vi "NEW LOAD CELL PID.vi"(5 "filtered_load_in":dbl, 6 "filtered_deriv_in":dbl, 7 "integral_out":dbl, 8 "error in (no error)":errorcluster, 9 "prev_error_out":dbl, 10 "Checkbox":bool, 11 "main ref":T1) -> (0 "error out":errorcluster, 1 "prev_error_out":dbl, 2 "integral_out":dbl, 3 "filtered_load_out":dbl, 4 "filtered_deriv_out":dbl)   [LabVIEW 2025]
uses:
  controls/LAB-IQ UI Data.ctl
  Traction Loop/Traction Receipe Enum.ctl
  HEAVE vi's/Heave Write enum.ctl
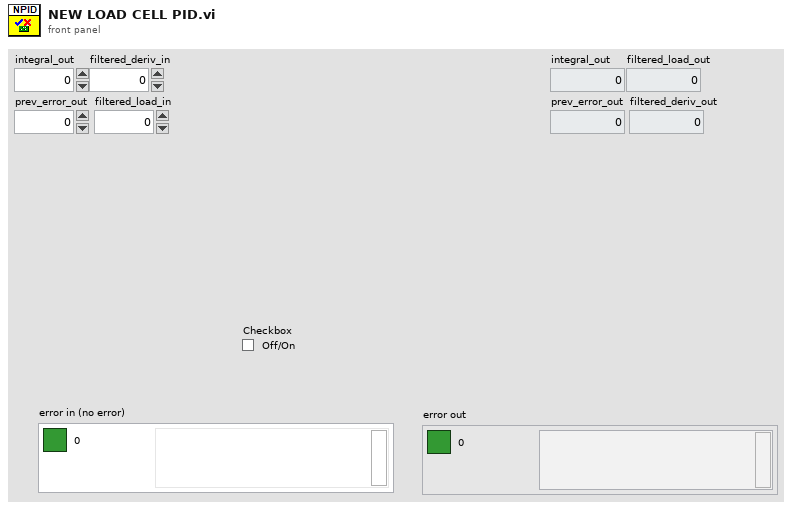
[diagram p1: front panel]
types:
  T1 = typedef "LAB-IQ UI Data.ctl" = cluster{"Main Home Screen":cluster{"GUI":refnum<vi>, "Platform Settings":refnum<vi>, "Configure":refnum<vi>, "Home":refnum<vi>, "EXIT":refnum<vi>, "service 2":refnum<vi>, "MainPage":refnum<vi>, "Analysis":refnum<vi>}, "Platform Settings":cluster{"mm/s  Surge":refnum<vi>, "Drive Error":refnum<vi>, "Disable Axis Jog Soft Limits":refnum<vi>, "mm/s  Sway":refnum<vi>, "Sway and Surge COM Status":refnum<vi>, "Heave COM Status":refnum<vi>, "Enable Platform":refnum<vi>, "Surge Forward Main":refnum<vi>, "Sway Right Main":refnum<vi>, "Sway Left Main":refnum<vi>, "Heave Down Main":refnum<vi>, "Heave Up main":refnum<vi>, "mm/s Heave":refnum<vi>, "mm/sec":refnum<vi>, "mm":refnum<vi>, "Surge Backward Main":refnum<vi>}, "Analysis Screen":cluster{"Analysis Home":refnum<vi>, "Surface Analysis":refnum<vi>, "Imaging":refnum<vi>, "Image Analysis":refnum<vi>, "Post Analysis":refnum<vi>}, "Config Screen":cluster{"Select Load Head":refnum<vi>, "Notes :":refnum<vi>, "FILE":refnum<vi>, "Sample ID :":refnum<vi>, "Operator ID :":refnum<vi>, "Operator Name :":refnum<vi>, "Auto":refnum<vi>}, "Motion Module":cluster{"zNL":refnum<vi>, "NL disp":refnum<vi>, "Rotary Tab":refnum<vi>, "Motion Direction:  3":refnum<vi>, "E.Velocity 2":refnum<vi>, "e.v/ssr 2":refnum<vi>, "Enter Fixed E.Velocity 2":refnum<vi>, "Enter Final SRR 2":refnum<vi>, "Enter initial SRR 2":refnum<vi>, "Enter Fixed SRR 2":refnum<vi>, "Enter the Final E.Velocity (m/s) 2":refnum<vi>, "Enter initial E.Velocity (m/s) 2":refnum<vi>, "Final Speed (RPM) 3":refnum<vi>, "Initial Speed (RPM) 2":refnum<vi>, "Enter the Final Velocity (m/s) 3":refnum<vi>, "Enter initial Velocity (m/s)  3":refnum<vi>, "Ramp Up 2":refnum<vi>, "TEST SELECTION":refnum<vi>, "SPEED SELECTION : ":refnum<vi>, "Angular Oscillation Set":refnum<vi>, "Traction":refnum<vi>, "Step Speed":refnum<vi>, "StepTable For Load-Speed":refnum<vi>, "StepTable For Speed":refnum<vi>, "Surge Forward MM":refnum<vi>, "Surge Backward MM":refnum<vi>, "M3 Image":refnum<vi>, "String 39":refnum<vi>, "Sway Left MM":refnum<vi>, "Sway Right MM":refnum<vi>, "Disable Axis Jog Soft Limits":refnum<vi>, "mm":refnum<vi>, "Heave Down MM":refnum<vi>, "Heave Up MM":refnum<vi>, "Wear Track Diameter (mm)":refnum<vi>, "Set WTD":refnum<vi>, "HomeScratch":refnum<vi>, "HomeRot":refnum<vi>, "PlaceModule":refnum<vi>, "Enter the Angle (Deg)":refnum<vi>, "Enter the Frequency (Hz)":refnum<vi>, "Motion Mode:":refnum<vi>, "LR Sway":refnum<vi>, "Rot Hor":refnum<vi>, "Scratch":refnum<vi>, "LR Cam":refnum<vi>, "MMBack":refnum<vi>, "MMNext":refnum<vi>, "Rot Ver":refnum<vi>, "Rotary Module Selection":refnum<vi>, "calculate rotary":refnum<vi>, "SPEED SELECTION : rotary":refnum<vi>, "Import 2":refnum<vi>, "Save 2":refnum<vi>, "File Path :  2":refnum<vi>, "String 45":refnum<vi>, "StepTable For Speed 3":refnum<vi>, "Enter the Speed(mm/sec)":refnum<vi>, "Enter the Speed(RPM)":refnum<vi>, "Enter Scratch Speed (mm/s):":refnum<vi>, "SwaySpeed Set":refnum<vi>, "Scartch Offset":refnum<vi>, "Motion type:":refnum<vi>, "HomeScratch 2":refnum<vi>, "Enter Scratch length (mm):":refnum<vi>, "Wear Track Diameter":refnum<vi>, "Rotary Speed Exced":refnum<vi>, "Scratch Mode":refnum<vi>, "No of Scratch":refnum<vi>}, "Environmental control":cluster{"Humidity  Status  3":refnum<vi>, "Low Temp  Status  2":refnum<vi>, "TK4 status 2":refnum<vi>, "Stage Temperature":refnum<vi>, "Sample Temperature":refnum<vi>, "Humidity (Amb)":refnum<vi>, "Clear List":refnum<vi>, "Add to list":refnum<vi>, "Wear":refnum<vi>, "Vibration":refnum<vi>, "Humidity (Chamber)":refnum<vi>, "Temperature (Chamber)":refnum<vi>, "ECR ":refnum<vi>, "Temperature (Amb)":refnum<vi>, "Microphone":refnum<vi>, "Acoustic Emission 3":refnum<vi>, "SNext":refnum<vi>, "APBack":refnum<vi>, "Enter the Temperature (°C):":refnum<vi>, "Enter the Stage \nTemperature (°C):":refnum<vi>, "Enter the Humidity (%Rh):":refnum<vi>, "Low Temp":refnum<vi>, "High Temp":refnum<vi>, "Humidity":refnum<vi>, "Sensors Picked":refnum<vi>}, "About Screen":cluster{"Password":refnum<vi>, "Home Service":refnum<vi>, "Advanced Setting":refnum<vi>, "About Tab":refnum<vi>, "ECR Port:":refnum<vi>, "Ramp Port:":refnum<vi>, "Installation/Replacement completed":refnum<vi>, "Loahead":refnum<vi>, "Heave and Surge COM Port:":refnum<vi>, "Sway COM Port:":refnum<vi>, "Temp Modbus:":refnum<vi>, "Humidity Port:":refnum<vi>, "Edit Gain Constants":refnum<vi>, "Save Gain Constants":refnum<vi>}, "Main Screen":cluster{"Main Screen Tab":refnum<vi>, "Angle and Frequency":refnum<vi>, "Stroke (mm)":refnum<vi>, "Angle (Deg)":refnum<vi>, "Main Speed Tab":refnum<vi>, "MTM MOTOR DISPLAY":refnum<vi>, "Disc Speed (m/sec)":refnum<vi>, "Ball Speed (m/sec)":refnum<vi>, "Disc Speed (RPM)":refnum<vi>, "Ball Speed (RPM)":refnum<vi>, "SPEED TAB":refnum<vi>, "Speed (m/sec)":refnum<vi>, "Set Speed (m/sec)":refnum<vi>, "Speed (RPM)":refnum<vi>, "Set Speed":refnum<vi>, "Time Tab":refnum<vi>, "Time ( HH:MM:SS ) 2":refnum<vi>, "Test Duration":refnum<vi>, "Test Duration 4":refnum<vi>, "TEST CYCLE":refnum<vi>, "TOTAL CYCLES":refnum<vi>, "Set Load (N)":refnum<vi>, "Temp Tabs":refnum<vi>, "Heater":refnum<vi>, "TK4 status":refnum<vi>, "ChamberTemp":refnum<vi>, "SetTmp":refnum<vi>, "Controller  Status":refnum<vi>, "ChamberTemp 2":refnum<vi>, "SetTmp 2":refnum<vi>, "Controller  Status 2":refnum<vi>, "ChamberTemp 3":refnum<vi>, "SetTmp 3":refnum<vi>, "Cooling":refnum<vi>, "Load Communication":refnum<vi>, "Ambient \nTemperature":refnum<vi>, "HumCOMStatus":refnum<vi>, "Ambient\n Humidity":refnum<vi>, "Freq (Hz)":refnum<vi>, "Load En":refnum<vi>, "NLt":refnum<vi>, "zNL 2":refnum<vi>, "Humidity On":refnum<vi>, "humidity disp":refnum<vi>, "Set Humidity":refnum<vi>, "NL disp 2":refnum<vi>, "Humidity On 2":refnum<vi>, "humidity disp 2":refnum<vi>, "Set Humidity 2":refnum<vi>, "NL disp 3":refnum<vi>, "AppLoadSeq scratch":refnum<vi>, "Stop Scratch":refnum<vi>, "ClrLog":refnum<vi>, "Trip Log":refnum<vi>, "STOP":refnum<vi>, "Start Test":refnum<vi>, "Test status":refnum<vi>, "AR Led":refnum<vi>, "Data":refnum<vi>, "Health":refnum<vi>, "Sway COM Status":refnum<vi>, "Heave COM Status":refnum<vi>, "Grp Tab":refnum<vi>, "Sub Graph":refnum<vi>, "SD (mm)":refnum<vi>, "Siliding distance Reset Graph":refnum<vi>, "SDGp":refnum<vi>, "Humidity Reset Graph":refnum<vi>, "HumrGp":refnum<vi>, "Acoustic Emission (mV)":refnum<vi>, "Aqucostic Reset Graph":refnum<vi>, "gACQUOS":refnum<vi>, "ECR RESET":refnum<vi>, "ECR":refnum<vi>, "Temperature Reset":refnum<vi>, "Acoustic Emission (mV) 2":refnum<vi>, "Aqucostic Reset Graph 2":refnum<vi>, "gACQUOS 2":refnum<vi>, "ECR RESET 2":refnum<vi>, "ECR 2":refnum<vi>, "Temperature Reset 2":refnum<vi>, "Temperature (deg c)":refnum<vi>, "Speed Reset Graph":refnum<vi>, "Speed Tab":refnum<vi>, "MTM DISC  SPEED":refnum<vi>, "MTM BALL SPEED":refnum<vi>, "speed mm/sec":refnum<vi>, "Hymidity":refnum<vi>, "Humidity Disable trip":refnum<vi>, "CoF Trip  2":refnum<vi>, "Depth Trip":refnum<vi>, "Weart Deapth":refnum<vi>, "Depth Reset Graph":refnum<vi>, "Weart":refnum<vi>, "Depthz":refnum<vi>, "Depth (µm)":refnum<vi>, "WearGp":refnum<vi>, "NL Trip 2":refnum<vi>, "Load pid":refnum<vi>, "Load Disable Trip":refnum<vi>, "Load Reset Graph":refnum<vi>, "NL Display 4":refnum<vi>, "Main Chart 3":refnum<vi>, "BACK":refnum<vi>, "Depth Trip 2":refnum<vi>, "COF TRIP ":refnum<vi>, "Friction Force (N)":refnum<vi>, "FF Reset Graph":refnum<vi>, "FF Disable Trip":refnum<vi>, "FF TRIP":refnum<vi>, "COF Disable Trip":refnum<vi>, "COF Reset Graph":refnum<vi>, "Start Test Temp":refnum<vi>, "zFF":refnum<vi>, "Friction Force (N) Graph":refnum<vi>, "Coefficient of Friction":refnum<vi>, "Scratch Start Test":refnum<vi>, "FF Tab":refnum<vi>, "Cyclic Friction Force (N)":refnum<vi>, "CZ FF":refnum<vi>, "Cyclic Friction Force (N) Graph":refnum<vi>, "Cyclic Coefficient of Friction":refnum<vi>, "Cyclic FF TRIP":refnum<vi>, "Cyclic FF Disable Trip":refnum<vi>, "cyclic COF Disable Trip":refnum<vi>, "cyclic COF TRIP":refnum<vi>, "cyclic COF Reset Graph":refnum<vi>, "Cyclic FF Reset Graph":refnum<vi>, "Test Trip":refnum<vi>, "Multi Scratch Pass":refnum<vi>, "Scratch Start Recording":refnum<vi>}, "Loading":cluster{"Indentation":refnum<vi>, "Reference Sample":refnum<vi>, "Load Cell Communication Slide":refnum<vi>, "com 3":refnum<vi>, "com":refnum<vi>, "DecaForce COM Status":refnum<vi>, "Update":refnum<vi>, "Clear 3":refnum<vi>, "seq":refnum<vi>, "Stribeck table":refnum<vi>, "Stribeck Table  For loading":refnum<vi>, "Loading Mode":refnum<vi>, "Enter the Final Load (N)":refnum<vi>, "Enter the CoF Trip":refnum<vi>, "Enter the Friction Force Trip":refnum<vi>, "Enter the Normal load Trip":refnum<vi>, "Enter the Load  (N)":refnum<vi>, "KiloForce":refnum<vi>, "DecaForce ":refnum<vi>, "MicroForce":refnum<vi>, "LHBack":refnum<vi>, "LHNext":refnum<vi>, "Enter the Loading Rate (N/min)":refnum<vi>, "Message":refnum<vi>, "Warning 2":refnum<vi>, "SSP 0.75":refnum<vi>, "SSP 0.5":refnum<vi>, "SSP 0.3":refnum<vi>, "Warning":refnum<vi>, "gui GIF":refnum<vi>, "Communication is established":refnum<vi>, "AppLoad 4":refnum<vi>, "Multipoint":refnum<vi>, "Load Selection":refnum<vi>}, "PID":cluster{"Ramp":refnum<vi>, "Vertical load (N)":refnum<vi>, "apply load":refnum<vi>, "apply load 2":refnum<vi>, "Enter ByPass Load":refnum<vi>, "Bypass Load":refnum<vi>, "gFF Rot":refnum<vi>}, "Config Parameters":cluster{"Tab Control 3":refnum<vi>, "Tab Control 19":refnum<vi>, "SAMPLES":refnum<vi>, "Re-initilaize":refnum<vi>, "Filter ON/OFF":refnum<vi>, "TracHomeSurgeOffsetCounts 10MM":refnum<vi>, "TracHomeSwayOffsetCounts 10MM":refnum<vi>, "Acoustic Emission:":refnum<vi>, "Apply Filter (FF)":refnum<vi>, "Filter% 2":refnum<vi>, "Apply Filter (Load)":refnum<vi>, "Filter% ":refnum<vi>, "Sway distance (mm)":refnum<vi>, "Surge distance (mm)":refnum<vi>, "DataSavingLoopDelay(ms)":refnum<vi>, "SAVE 2":refnum<vi>, "Enter Distance":refnum<vi>, "Sway Counts:":refnum<vi>, "Distance (mm): 3":refnum<vi>, "Surge Counts:":refnum<vi>, "Distance (mm): 2":refnum<vi>, "Distance (mm):":refnum<vi>, "Heave Counts:":refnum<vi>, "LRMHomeSurgeOffsetCounts":refnum<vi>, "LRMHomeSwayOffsetCounts":refnum<vi>, "TracHomeSurgeOffsetCounts 20MM":refnum<vi>, "TracHomeSwayOffsetCounts 20MM":refnum<vi>, "RotHomeSwayOffsetCounts":refnum<vi>, "RotHomeSurgeOffsetCounts":refnum<vi>, "Heave distance":refnum<vi>, "Zmm":refnum<vi>, "Heave Pulses/mm":refnum<vi>, "Surge Pulses/mm":refnum<vi>, "Sway Pulses/mm":refnum<vi>, "Heave Pitch":refnum<vi>, "Surge Pitch":refnum<vi>, "Sway Pitch":refnum<vi>, "Heave PPR":refnum<vi>, "Surge PPR":refnum<vi>, "Sway PPR":refnum<vi>, "Tab Control 5":refnum<vi>, "Tab Control 14":refnum<vi>, "Tab Control 26":refnum<vi>, "AE":refnum<vi>, "Heave Loop Delay":refnum<vi>, "Heave PID Speed":refnum<vi>, "Surge Jog Speed":refnum<vi>, "Heave Jog Speed":refnum<vi>, "Sway Loop Delay":refnum<vi>, "Sway PID Speed":refnum<vi>, "Sway Jog Speed":refnum<vi>, "DEPTH TRIP VALUE":refnum<vi>, "LOAD TRIP VALUE":refnum<vi>, "DEPTH TRIP   ENABLE":refnum<vi>, "LOAD TRIP  ENABLE":refnum<vi>, "CYCLIC FF TRIP VALUE":refnum<vi>, "FF TRIP VALUE":refnum<vi>, "CYCLIC CoF TRIP VALUE":refnum<vi>, "COF TRIP VALUE":refnum<vi>, "CYCLIC COF TRIP  ENABLE":refnum<vi>, "CYCLIC FF TRIP  ENABLE":refnum<vi>, "FF TRIP  ENABLE":refnum<vi>, "COF TRIP  ENABLE":refnum<vi>, "JOG TRIP LOAD VALUE (N)":refnum<vi>, "Rotary Vertical":refnum<vi>, "Traction":refnum<vi>, "Scratch":refnum<vi>, "LRM CAM":refnum<vi>, "Sway LRM":refnum<vi>, "Rotary Horizontal":refnum<vi>}, "Loading Com Port":cluster{"ClearAll":refnum<vi>, "Mz(Nm)":refnum<vi>, "My(Nm)":refnum<vi>, "Mx(Nm)":refnum<vi>, "Save Dwell":refnum<vi>, "Acq Delay (ms)":refnum<vi>, "Burst Delay (ms)":refnum<vi>, "model":refnum<vi>, "SN":refnum<vi>, "FFx(N)":refnum<vi>, "Sensor IP":refnum<vi>, "Port":refnum<vi>, "FFy(N)":refnum<vi>, "Load(N)":refnum<vi>, "delete Handle":refnum<vi>, "Create Handle":refnum<vi>, "ft_data":refnum<vi>, "ft_range":refnum<vi>, "ft_data 2":refnum<vi>, "stop 6":refnum<vi>, "running_flag":refnum<vi>, "ft_udp_handle":refnum<vi>, "get-data-return":refnum<vi>, "get-range-return":refnum<vi>, "zero-return":refnum<vi>, "filter-return":refnum<vi>, "initial-return":refnum<vi>, "deleteHandle-result":refnum<vi>, "Load Cell Temp":refnum<vi>, "Load Cell":refnum<vi>, "ZeroAll":refnum<vi>, "FORCE (N)":refnum<vi>, "TORQUE (N-m)":refnum<vi>, "Load Cell Link":refnum<vi>}, "Heave AND Surge":cluster{"SURGE POSE":refnum<vi>, "error out Read":refnum<vi>, "HEAVE POSE":refnum<vi>, "State":refnum<vi>, "Homed":refnum<vi>, "Sequence ID":refnum<vi>, "error out Write":refnum<vi>, "faultCode":refnum<vi>, "Ack ID":refnum<vi>, "SPEED":refnum<vi>, "Distance":refnum<vi>, "Mode Command":refnum<vi>, "Heave and Surge Read":refnum<vi>, "Read Heave Temp":refnum<vi>, "Spare 15":refnum<vi>, "Spare 14":refnum<vi>, "Spare 13":refnum<vi>, "Spare 12":refnum<vi>, "Spare 11":refnum<vi>, "Spare 10":refnum<vi>, "Spare 9":refnum<vi>, "Spare 8":refnum<vi>, "Spare 7":refnum<vi>, "Spare 4":refnum<vi>, "Spare 3":refnum<vi>, "Spare 2":refnum<vi>, "Humidity":refnum<vi>, "Temp":refnum<vi>, "Node Id":refnum<vi>, "Spare 1":refnum<vi>, "SPARE 4":refnum<vi>, "SPARE 3":refnum<vi>, "SPARE 2":refnum<vi>, "SPARE 1":refnum<vi>, "fwMajor":refnum<vi>, "fwMinor":refnum<vi>, "Manual Write":refnum<vi>, "Heave and Surge Write":refnum<vi>, "SPARE 5":refnum<vi>, "Reserved ":refnum<vi>, "SPARE 8":refnum<vi>, "SPARE 6":refnum<vi>, "SPARE 7":refnum<vi>, "SPARE 17":refnum<vi>, "SPARE 16":refnum<vi>, "SPARE 15":refnum<vi>, "SPARE 14":refnum<vi>, "SPARE 13":refnum<vi>, "SPARE 12":refnum<vi>, "SPARE 11":refnum<vi>, "SPARE 10":refnum<vi>, "SPARE 9":refnum<vi>, "System UPTIME":refnum<vi>, "Missed Packets":refnum<vi>, "faultCode Surge Right":refnum<vi>, "faultCode Surge Left":refnum<vi>, "faultCode Heave":refnum<vi>, "UPLINK HEAVE":refnum<vi>, "DOWNLINK HEAVE":refnum<vi>}, "New PID LOGIC":cluster{"Fine Tune Zone":refnum<vi>, "PID SDelay":refnum<vi>, "Max_pos_limit":refnum<vi>, "Min_pos_limit":refnum<vi>, "i_limit":refnum<vi>, "pct_scale":refnum<vi>, "Deadband":refnum<vi>, "Kd":refnum<vi>, "Ki":refnum<vi>, "Kp":refnum<vi>, "Current Position":refnum<vi>, "Set Load":refnum<vi>, "Current Load":refnum<vi>, "Pulse delta":refnum<vi>, "Init Step":refnum<vi>, "Max Step Linit":refnum<vi>, "min_deadband_floor":refnum<vi>, "dynamic_spindle_noise_scalar":refnum<vi>, "min_finetune_floor":refnum<vi>, "filter_alpha":refnum<vi>, "PID":refnum<vi>}, "SWAY ":cluster{"fwMajor":refnum<vi>, "Homed":refnum<vi>, "Rotary POSE":refnum<vi>, "State":refnum<vi>, "SWAY POSE":refnum<vi>, "Ack ID":refnum<vi>, "faultCode":refnum<vi>, "Node Id":refnum<vi>, "fwMinor":refnum<vi>, "Spare 6":refnum<vi>, "Spare 5":refnum<vi>, "Spare 4":refnum<vi>, "Spare 3":refnum<vi>, "Spare 2":refnum<vi>, "Spare 1":refnum<vi>, "Spare 7":refnum<vi>, "SPARE  5":refnum<vi>, "error out Write  SWAY ":refnum<vi>, "error out Read SWAY ":refnum<vi>, "Manual Write SWAY ":refnum<vi>, "SWAY WRITE":refnum<vi>, "SPARE  4":refnum<vi>, "SPARE  3":refnum<vi>, "SPARE 2":refnum<vi>, "SPARE 1":refnum<vi>, "Spare 15":refnum<vi>, "Spare 14":refnum<vi>, "Spare 13":refnum<vi>, "Spare 12":refnum<vi>, "Spare 11":refnum<vi>, "Spare 9":refnum<vi>, "Spare 8":refnum<vi>, "SPEED":refnum<vi>, "Distance":refnum<vi>, "Mode Command":refnum<vi>, "Sequence ID":refnum<vi>, "SWAY READ":refnum<vi>, "Spare 10":refnum<vi>, "Read SWAY Temp":refnum<vi>, "faultCode Sway ":refnum<vi>, "Missed Packets":refnum<vi>, "System UPTIME sway":refnum<vi>, "SPARE 6":refnum<vi>, "SPARE 7":refnum<vi>, "SPARE 9":refnum<vi>, "SPARE 11":refnum<vi>, "SPARE 10":refnum<vi>, "SPARE 8":refnum<vi>, "SPARE 13":refnum<vi>, "SPARE 12":refnum<vi>, "SPARE 17":refnum<vi>, "SPARE 16":refnum<vi>, "SPARE 15":refnum<vi>, "SPARE 14":refnum<vi>, "Reserved":refnum<vi>, "faultCode Rotary":refnum<vi>, "UPLINK SWAY":refnum<vi>, "DOWNLINK SWAY":refnum<vi>}, "Analysis Screen":cluster{"Analysis Home":refnum<vi>, "Refresh 2":refnum<vi>, "MEAN 4":refnum<vi>, "SD 4":refnum<vi>, "VARIANCE 4":refnum<vi>, "MEAN  3":refnum<vi>, "SD  3":refnum<vi>, "VARIANCE  3":refnum<vi>, "MEAN 2":refnum<vi>, "SD  2":refnum<vi>, "VARIANCE 2":refnum<vi>, "MEAN":refnum<vi>, "SD":refnum<vi>, "VARIANCE":refnum<vi>, "File 4 Discription":refnum<vi>, "OPEN 4":refnum<vi>, "File Name 4":refnum<vi>, "OPEN 3":refnum<vi>, "File 3 Discription":refnum<vi>, "File Name 3":refnum<vi>, "Y-AXIS":refnum<vi>, "X-AXIS":refnum<vi>, "XY Graph":refnum<vi>, "File Name 2":refnum<vi>, "File Name 1":refnum<vi>, "OPEN 2":refnum<vi>, "OPEN 1":refnum<vi>, "File 1 Discription ":refnum<vi>, "File 2 Discription":refnum<vi>, "Export":refnum<vi>, "File Format":refnum<vi>}, "Traction":cluster{"faultCode Traction 2":refnum<vi>, "faultCode Traction 1":refnum<vi>, "Missed Packets":refnum<vi>, "System UPTIME Traction":refnum<vi>, "SPARE 17":refnum<vi>, "SPARE 16":refnum<vi>, "SPARE 15":refnum<vi>, "SPARE 14":refnum<vi>, "SPARE 13":refnum<vi>, "SPARE 12":refnum<vi>, "SPARE 11":refnum<vi>, "SPARE 10":refnum<vi>, "SPARE 9":refnum<vi>, "SPARE 8":refnum<vi>, "SPARE 7":refnum<vi>, "SPARE 6":refnum<vi>, "Reserved":refnum<vi>, "SPARE  5":refnum<vi>, "Manual Write TRACTION":refnum<vi>, "TRACTION WRITE":refnum<vi>, "SPARE  4":refnum<vi>, "SPARE  3":refnum<vi>, "SPARE 2":refnum<vi>, "SPARE 1":refnum<vi>, "Spare 7":refnum<vi>, "Spare 6":refnum<vi>, "Spare 5":refnum<vi>, "Spare 4":refnum<vi>, "Spare 2":refnum<vi>, "Spare 1":refnum<vi>, "Node Id":refnum<vi>, "Read TRACTION Temp":refnum<vi>, "fwMinor":refnum<vi>, "fwMajor":refnum<vi>, "faultCode":refnum<vi>, "TRACTION POSE":refnum<vi>, "TRACTION POSE 2":refnum<vi>, "Homed":refnum<vi>, "State":refnum<vi>, "Ack ID":refnum<vi>, "SPEED":refnum<vi>, "Distance":refnum<vi>, "Mode Command":refnum<vi>, "Sequence ID":refnum<vi>, "error out Read TRACTION":refnum<vi>, "error out Write  TRACTION":refnum<vi>, "TRACTION READ":refnum<vi>, "Spare 3":refnum<vi>, "Downlink traction":refnum<vi>, "Uplink Traction":refnum<vi>}, "Traction reciepe":cluster{"SRR Sweep Range (%) Stribeck":refnum<vi>, "Traction Receipe":refnum<vi>, "Total Execution Time":refnum<vi>, "Total Steps":refnum<vi>, "Duration / Step (s)  Stribeck":refnum<vi>, "STRIBECK Fixed SRR List (%)":refnum<vi>, "Duration / Step (s) Traction":refnum<vi>, "SRR Sweep Range (%) traction":refnum<vi>, "Rolling Speed (mm/s)":refnum<vi>, "Temperature Stages (°C)":refnum<vi>, "Ball Load (N)":refnum<vi>, "Lubricant Name":refnum<vi>, "Profile File Name":refnum<vi>, "SET entrainment Velocity":refnum<vi>, "Test Array Size":refnum<vi>, "SRR INDEX [ STRIBECK]":refnum<vi>, "Stribeck Size":refnum<vi>, "SET SRR":refnum<vi>, "ELAPSED TIMER ":refnum<vi>, "BALL SET RPM":refnum<vi>, "DISC SET RPM":refnum<vi>, "SET LOAD":refnum<vi>, "TEMPERATURE READ":refnum<vi>, "SET TEMPERATURE":refnum<vi>, "Traction Size":refnum<vi>, "DISC SPEED (rpm)":refnum<vi>, "BALL SPEED (rpm)":refnum<vi>, "BALL WEAR TRACK":refnum<vi>, "DISC WEARTRACK":refnum<vi>, "SRR INDEX [ TRACTION]":refnum<vi>, "Start Index Type":refnum<vi>, "Enum - Menu":refnum<vi>, "Ball (mm/sec)":refnum<vi>, "Disc (mm/sec)":refnum<vi>}, "Traction Control":cluster{"HomeTraction":refnum<vi>, "Demo Mode Display":refnum<vi>, "Traction Message":refnum<vi>, "Traction Step Update Details":refnum<vi>, "Main Tab sequence for selection":refnum<vi>, "Ramp Tab":refnum<vi>, "e.v/ssr":refnum<vi>, "Enter Fixed E.Velocity":refnum<vi>, "Enter Final SRR":refnum<vi>, "Enter initial SRR":refnum<vi>, "Enter Fixed SRR":refnum<vi>, "Enter the Final E.Velocity (m/s)":refnum<vi>, "Enter initial E.Velocity (m/s)":refnum<vi>, "Ball WTD":refnum<vi>, "E.Velocity":refnum<vi>, "Enter the Final Velocity (m/s)":refnum<vi>, "Enter initial Velocity (m/s)":refnum<vi>, "Ramp Up   Disc":refnum<vi>, "Initial DiscSpeed (RPM)":refnum<vi>, "Final Speed (RPM) Ball":refnum<vi>, "Final Speed (RPM)":refnum<vi>, "Initial Speed (RPM) Ball":refnum<vi>, "Enter the Final Velocity (m/s) Ball":refnum<vi>, "Enter initial Velocity (m/s) Ball":refnum<vi>, "Ramp Up":refnum<vi>, "ExceedBallSpeed step":refnum<vi>, "ExceedDiscSpeed":refnum<vi>, "BallSpeed Exceed Indication":refnum<vi>, "Apply":refnum<vi>, "SPEED SELECTION : MTM":refnum<vi>, "SPEED SELECTION : MTM 2":refnum<vi>, "TEST SELECTION (MTM)":refnum<vi>, "MTM Test Selection":refnum<vi>, "File Path Tab":refnum<vi>, "File Path String":refnum<vi>, "Save":refnum<vi>, "Save  2":refnum<vi>, "Import ":refnum<vi>, "File Path :":refnum<vi>, "Step Sequence Indication Tab":refnum<vi>, "Step Sequence Indication":refnum<vi>, "Calculate Step":refnum<vi>, "StepTable":refnum<vi>, "ExceedDiscSpeed  Cinstant Speed":refnum<vi>, "ExceedBallSpeed Constant":refnum<vi>, "TEST SELECTION (MTM) 2":refnum<vi>, "SPEED SELECTION : MTM 3":refnum<vi>, "MTM Test Selection 2":refnum<vi>, "Enter the Speed (m/sec): ":refnum<vi>, "Enter the Speed (m/sec):  2":refnum<vi>, "Enter the Speed (RPM):":refnum<vi>, "Lower Spped ":refnum<vi>, "Upper":refnum<vi>, "Enter the Speed (RPM):Ball":refnum<vi>, "Disc Motion Direction: ":refnum<vi>, "Ball Motion Direction :":refnum<vi>, "Motion Mode: ":refnum<vi>, "Wear Track Diameter (mm) ":refnum<vi>, "Disc Speed Indicator":refnum<vi>, "ExceedBallSpeed":refnum<vi>}, "Acquostic":cluster{"Last Config Rejected ":refnum<vi>, "rx command count":refnum<vi>, "Current Filter Id":refnum<vi>, "Isolated Gain":refnum<vi>, "DAQ Status":refnum<vi>, "error out":refnum<vi>, "error in (no error)":refnum<vi>, "Uplink Packet":refnum<vi>, "data out":refnum<vi>, "Downlink Packet":refnum<vi>, "Gains":refnum<vi>, "Manual Write Acquostic":refnum<vi>, "Acoustic Graphs":refnum<vi>}}
  T2 = cluster{"min_deadband_floor":dbl, "min_finetune_floor":dbl, "dynamic_spindle_noise_scalar":dbl, "filter_alpha":dbl, "Vertical load (N)":dbl, "Pulse delta":dbl, "Fine Tune Zone":dbl, "Max_pos_limit":dbl, "Min_pos_limit":dbl, "i_limit":dbl, "Max Step Linit":dbl, "Init Step":dbl, "pct_scale":dbl, "Deadband":dbl, "Kd":dbl, "Ki":dbl, "Kp":dbl, "Current Position":dbl, "Set Load":dbl, "Current Load":dbl, "gFF Rot 7":cluster{dbl, dbl, dbl}, "Bypass Load":bool, "Enter ByPass Load":dbl, "apply load":bool}
  T3 = cluster{"Sequence ID":u16, "Mode Command":u8, "Distance":sgl, "SPEED":sgl, "Reserved":sgl, "SPARE 1":u8, "SPARE 2":u8, "SPARE 3":u8, "SPARE 4":u8, "SPARE 5":u8, "SPARE 6":u8, "SPARE 7":u8, "SPARE 8":u8, "SPARE 9":u8, "SPARE 10":u8, "SPARE 11":u8, "SPARE 12":u8, "SPARE 13":u8, "SPARE 14":u8, "SPARE 15":u8, "SPARE 16":u8, "SPARE 17":u8}
  T4 = typedef "Heave Write enum.ctl" = enum16{"INIT", "WRITE", "CLOSE", "REINIT"}
  T5 = cluster{"Ack ID":u16, "State":u8, "Homed":u8, "HEAVE POSE":sgl, "SURGE POSE":sgl, "faultCode":u16, "fwMajor":u8, "fwMinor":u8, "Node Id":u8, "Spare 1":u8, "Spare 2":u8, "Spare 3":u8, "Spare 4":u8, "Spare 5":u8, "Spare 6":u8, "Spare 7":u8, "System UPTIME":sgl, "Missed Packets":sgl, "faultCode Heave":u16, "faultCode Surge Left":u16, "faultCode Surge Right":u16}
  T6 = cluster{"Value":dbl, "Vertical load (N)":dbl, dbl}
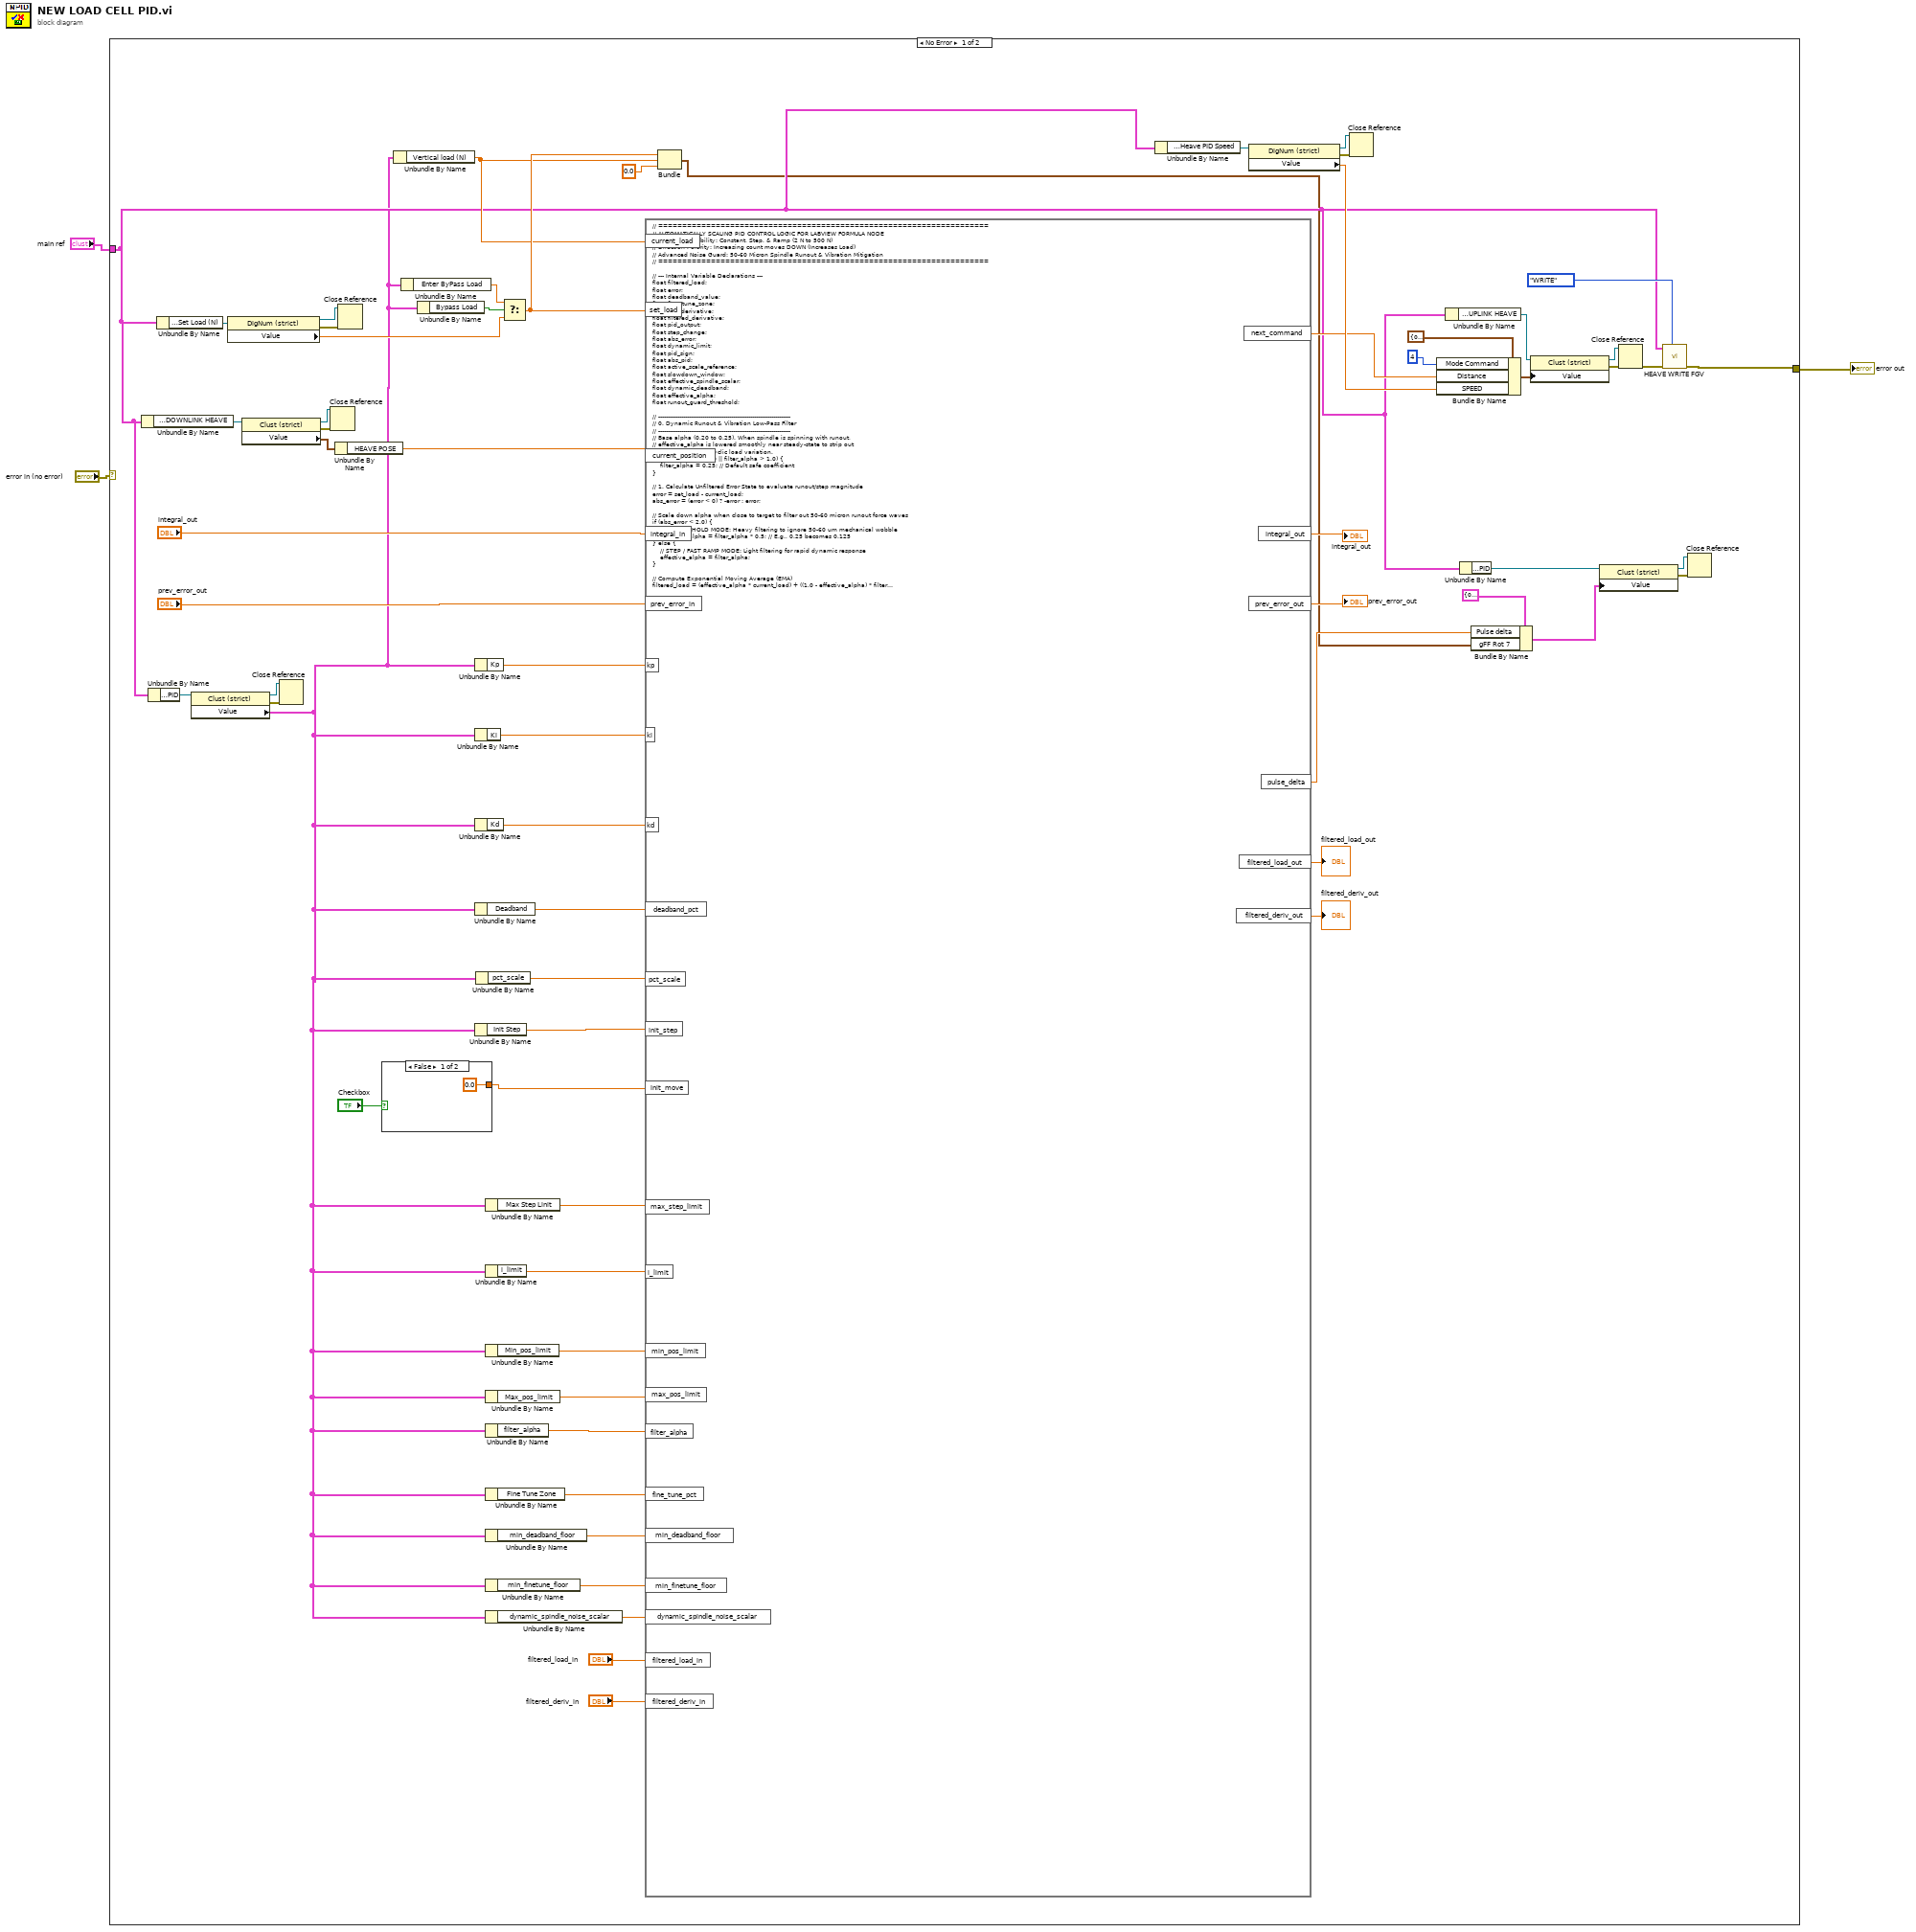
[diagram p0: block diagram]
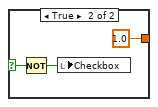
[diagram p2: hidden frame]
diagram:
  n1 = case shown="No Error" "error in (no error)" {
    tunnel: "main ref" -> [w10 _]
    tunnel: [w68 _] -> w1
    frame No Error {
      n2 = Unbundle By Name(w10) -> ("Heave AND Surge.DOWNLINK HEAVE"=w36:refnum<vi>)
      n3 = Unbundle By Name(w10) -> ("New PID LOGIC.PID"=w31:refnum<vi>)
      n4 = Unbundle By Name(w10) -> ("Main Screen.Set Load (N)"=w63:refnum<vi>)
      n5 = property on="Property Node" class="Clust (strict)"(reference=w31) -> (reference out=w33:refnum<vi>, error out=w32:errorcluster, "Value"=w5:T2)  [unwired: 1 in]
      n6 = property class="DigNum (strict)"(reference=w63) -> (reference out=w65:refnum<vi>, error out=w64:errorcluster, "Value"=w62:dbl)  [unwired: 1 in]
      n7 = property on="Property Node" class="Clust (strict)"(reference=w36) -> (reference out=w38:refnum<vi>, error out=w37:errorcluster, "Value"=w35:T5)  [unwired: 1 in]
      n8 = Close Reference(reference=w33, error in (no error)=w32) -> ()  [unwired: 1 out]
      n9 = Close Reference(reference=w38, error in (no error)=w37) -> ()  [unwired: 1 out]
      n10 = Unbundle By Name(w35) -> ("HEAVE POSE"=w34:sgl)
      n11 = Close Reference(reference=w65, error in (no error)=w64) -> ()  [unwired: 1 out]
      n12 = case shown="False" "Checkbox" {
        selector: "Checkbox" -> [_ w72]
        tunnel: [0.0 1.0] -> w60
        frame False {
        }
        frame True {
          n13 = Not(x=w72) -> (.not. x?=w71:bool)
          n14 = local write "Checkbox"(w71) -> ()
        }
      }
      n15 = Unbundle By Name(w5) -> ("Vertical load (N)"=w14:dbl)
      n16 = Unbundle By Name(w5) -> ("Enter ByPass Load"=w15:dbl)
      n17 = Unbundle By Name(w5) -> ("Bypass Load"=w16:bool)
      n18 = Unbundle By Name(w5) -> ("Kp"=w30:dbl)
      n19 = Unbundle By Name(w5) -> ("Ki"=w29:dbl)
      n20 = Unbundle By Name(w5) -> ("Kd"=w28:dbl)
      n21 = Unbundle By Name(w5) -> ("Deadband"=w27:dbl)
      n22 = Unbundle By Name(w5) -> ("Init Step"=w4:dbl)
      n23 = Unbundle By Name(w5) -> ("pct_scale"=w26:dbl)
      n24 = Unbundle By Name(w5) -> ("Max Step Linit"=w25:dbl)
      n25 = Unbundle By Name(w5) -> ("i_limit"=w24:dbl)
      n26 = Unbundle By Name(w5) -> ("Min_pos_limit"=w23:dbl)
      n27 = Unbundle By Name(w5) -> ("Max_pos_limit"=w22:dbl)
      n28 = Unbundle By Name(w5) -> ("filter_alpha"=w21:dbl)
      n29 = Unbundle By Name(w5) -> ("Fine Tune Zone"=w20:dbl)
      n30 = Unbundle By Name(w5) -> ("min_deadband_floor"=w19:dbl)
      n31 = Unbundle By Name(w5) -> ("min_finetune_floor"=w18:dbl)
      n32 = Unbundle By Name(w5) -> ("dynamic_spindle_noise_scalar"=w17:dbl)
      n33 = Select(t=w15, s=w16, f=w62) -> (s? t:f=w52:dbl)
      n34 = formula code="// =====================================================================\n// AUTOMATICALLY SCALING PID CONTROL LOGIC FOR LABVIEW FORMULA NODE\n// Profile Adaptability: Constant, Step, & Ramp (2 N to 500 N)\n// Direction Polarity: Increasing count moves DOWN (Increases Load)\n// Advanced Noise Guard: 50-60 Micron Spindle Runout & Vibration Mitigation\n// =====================================================================\n\n// --- Internal Variable Declarations ---\nfloat filtered_load;\nfloat error;\nfloat deadband_value;\nfloat fine_tune_zone;\nfloat raw_derivative;\nfloat filtered_derivative;\nfloat pid_output;\nfloat step_change;\nfloat abs_error;\nfloat dynamic_limit;\nfloat pid_sign;\nfloat abs_pid;\nfloat active_scale_reference;\nfloat slowdown_window;\nfloat effective_spindle_scalar;\nfloat dynamic_deadband;\nfloat effective_alpha;\nfloat runout_guard_threshold;\n\n// ---------------------------------------------------------------------\n// 0. Dynamic Runout & Vibration Low-Pass Filter\n// ---------------------------------------------------------------------\n// Base alpha (0.20 to 0.25). When spindle is spinning with runout, \n// effective_alpha is lowered smoothly near steady-state to strip out \n// the 50-60 micron cyclic load variation.\nif (filter_alpha <= 0.0 || filter_alpha > 1.0) {\n    filter_alpha = 0.25; // Default safe coefficient\n}\n\n// 1. Calculate Unfiltered Error State to evaluate runout/step magnitude\nerror = set_load - current_load;\nabs_error = (error < 0) ? -error : error;\n\n// Scale down alpha when close to target to filter out 50-60 micron runout force waves\nif (abs_error < 2.0) {\n    // RUNOUT HOLD MODE: Heavy filtering to ignore 50-60 um mechanical wobble\n    effective_alpha = filter_alpha * 0.5; // E.g., 0.25 becomes 0.125\n} else {\n    // STEP / FAST RAMP MODE: Light filtering for rapid dynamic response\n    effective_alpha = filter_alpha; \n}\n\n// Compute Exponential Moving Average (EMA)\nfiltered_load = (effective_alpha * current_load) + ((1.0 - effective_alpha) * filtered_load_in);\nfiltered_load_out = filtered_load; // Output to feedback shift register\n\n// Recalculate Error using Filtered Load\nerror = set_load - filtered_load;\nabs_error = (error < 0) ? -error : error;\n\n// 2. Establish Scale Reference (Safeguards low-load ramp profiles)\nactive_scale_reference = (set_load < 2.0) ? 2.0 : set_load;\n\n// 3. Dynamic & Ramp-Safe Deadband Calculation (Runout Absorber)\n// Accounts for physical load ripple caused by 50-60 micron disc runout\nrunout_guard_threshold = 1.5; // Newton threshold where move is considered dynamic\n\nif (abs_error > runout_guard_threshold) {\n    effective_spindle_scalar = 0.0; // RAMP/STEP MODE: Zero deadband expansion\n} else {\n    // HOLD MODE: Expand deadband slightly to absorb 50-60 um runout force amplitude\n    effective_spindle_scalar = dynamic_spindle_noise_scalar; \n}\n\ndynamic_deadband = deadband_pct * (1.0 + effective_spindle_scalar); \n\ndeadband_value = active_scale_reference * (dynamic_deadband / pct_scale);\nif (deadband_value < 0) {\n    deadband_value = -deadband_value; \n}\nif (deadband_value < min_deadband_floor) {\n    deadband_value = min_deadband_floor; \n}\n\n// 4. Compute Dynamic Fine-Tune Zone with Floor Guard\nfine_tune_zone = active_scale_reference * (fine_tune_pct / pct_scale);\nif (fine_tune_zone < 0) {\n    fine_tune_zone = -fine_tune_zone;\n}\nif (fine_tune_zone < min_finetune_floor) {\n    fine_tune_zone = min_finetune_floor;\n}\n\n// 5. Main Control State Machine\n// ---------------------------------------------------------------------\n// Condition A: Initial Move (Establish baseline and force initial step)\n// ---------------------------------------------------------------------\nif (init_move == 1) {\n    step_change = init_step; \n    integral_out = 0.0;                 // Reset integral memory\n    prev_error_out = error;             // Initialize derivative baseline\n    filtered_deriv_out = 0.0;           // Reset derivative filter memory\n    \n    if (error > 0) {\n        next_command = current_position + step_change;\n    } else {\n        next_command = current_position - step_change;\n    }\n    pulse_delta = next_command - current_position;\n}\n// ---------------------------------------------------------------------\n// Condition B: Within Target Deadband (Freeze State / Suppress Runout Hunting)\n// ---------------------------------------------------------------------\nelse if (abs_error <= deadband_value) {\n    step_change = 0.0;\n    next_command = current_position;  // Lock physical position\n    integral_out = integral_in;        // Freeze integral to prevent runout windup\n    prev_error_out = error;            // Keep derivative baseline fresh\n    filtered_deriv_out = 0.0;          // Zero derivative output\n    pulse_delta = 0.0;                 // Zero motor pulse energy completely\n} \n// ---------------------------------------------------------------------\n// Condition C: Active PID Control Zone (Step, Ramp, & Active Adjustment)\n// ---------------------------------------------------------------------\nelse {\n    // A. Anti-Windup Integral Action (Freezes integral if oscillating close to target)\n    if (abs_error <= (deadband_value * 1.5)) {\n        integral_out = integral_in; // Freeze integral in near-deadband zone to prevent runout windup\n    } else {\n        integral_out = integral_in + error;\n        if (integral_out > i_limit) {\n            integral_out = i_limit;\n        } else if (integral_out < -i_limit) {\n            integral_out = -i_limit;\n        }\n    }\n\n    // B. Low-Pass Filtered Derivative Action\n    // Eliminates high-frequency derivative spikes caused by 50-60 um disc runout\n    raw_derivative = error - prev_error_in;\n    prev_error_out = error;\n\n    filtered_derivative = (0.20 * raw_derivative) + (0.80 * filtered_deriv_in);\n    filtered_deriv_out = filtered_derivative; \n\n    // C. Execute Filtered PID Calculation\n    pid_output = (error * kp) + (integral_out * ki) + (filtered_derivative * kd);\n    \n    // D. Extract Mathematical Sign and Magnitude\n    pid_sign = (pid_output >= 0) ? 1.0 : -1.0;\n    abs_pid = (pid_output < 0) ? -pid_output : pid_output;\n\n    // E. Continuous Linear Ramp-Down Ceiling\n    slowdown_window = 2.0; \n\n    if (abs_error < slowdown_window) {\n        dynamic_limit = max_step_limit * (abs_error / slowdown_window);\n        if (dynamic_limit < 1.0) {\n            dynamic_limit = 1.0; \n        }\n    } else {\n        dynamic_limit = max_step_limit; \n    }\n\n    // F. Apply Smooth Step Control & Fine Tuning Zone\n    if (abs_error <= 0.5) {\n        step_change = 1.0; \n    } else {\n        if (abs_pid < dynamic_limit) {\n            step_change = abs_pid; \n        } else {\n            step_change = dynamic_limit; \n        }\n    }\n    \n    // G. Minimum Physical Pulse Guard\n    if (step_change < 1.0) {\n        step_change = 1.0;\n    }\n    \n    // H. Apply Step Vector\n    next_command = current_position + (step_change * pid_sign);\n    pulse_delta = next_command - current_position;\n}\n\n// 6. Hard Structural Boundaries & Safety Guards\n// ---------------------------------------------------------------------\nif (next_command > max_pos_limit) {\n    next_command = max_pos_limit;\n    pulse_delta = next_command - current_position;\n} else if (next_command < min_pos_limit) {\n    next_command = min_pos_limit;\n    pulse_delta = next_command - current_position;\n}"("current_load"=w14, "set_load"=w52, "current_position"=w34, "integral_in"="integral_out", "prev_error_in"="prev_error_out", "kp"=w30, "ki"=w29, "kd"=w28, "deadband_pct"=w27, "pct_scale"=w26, "init_step"=w4, "init_move"=w60, "max_step_limit"=w25, "i_limit"=w24, "min_pos_limit"=w23, "max_pos_limit"=w22, "fine_tune_pct"=w20, "min_deadband_floor"=w19, "min_finetune_floor"=w18, "filter_alpha"=w21, "dynamic_spindle_noise_scalar"=w17, "filtered_load_in"="filtered_load_in", "filtered_deriv_in"="filtered_deriv_in") -> ("next_command"=w39:dbl, "integral_out"=→"integral_out":dbl, "prev_error_out"=→"prev_error_out":dbl, "pulse_delta"=w7:dbl, "filtered_load_out"=→"filtered_load_out":dbl, "filtered_deriv_out"=→"filtered_deriv_out":dbl)
      n35 = Bundle("Value"=w52, "Vertical load (N)"=w14, 0.0) -> (w6:T6)  [unwired: 1 in]
      n36 = Unbundle By Name(w10) -> ("Config Parameters.Heave PID Speed"=w55:refnum<vi>)
      n37 = property class="DigNum (strict)"(reference=w55) -> (reference out=w57:refnum<vi>, error out=w56:errorcluster, "Value"=w40:dbl)  [unwired: 1 in]
      n38 = Close Reference(reference=w57, error in (no error)=w56) -> ()  [unwired: 1 out]
      n39 = Bundle By Name(cluster=T3 {"Sequence ID"=0, "Mode Command"=0, "Distance"=0.0, "SPEED"=0.0, "Reserved"=0.0, "SPARE 1"=0, "SPARE 2"=0, "SPARE 3"=0, "SPARE 4"=0, "SPARE 5"=0, "SPARE 6"=0, "SPARE 7"=0, "SPARE 8"=0, "SPARE 9"=0, "SPARE 10"=0, "SPARE 11"=0, "SPARE 12"=0, "SPARE 13"=0, "SPARE 14"=0, "SPARE 15"=0, "SPARE 16"=0, "SPARE 17"=0} ("Value"), "Mode Command"=u8 4, "Distance"=w39, "SPEED"=w40) -> (w47:T3)
      n40 = Unbundle By Name(w10) -> ("Heave AND Surge.UPLINK HEAVE"=w42:refnum<vi>)
      n41 = Unbundle By Name(w10) -> ("New PID LOGIC.PID"=w11:refnum<vi>)
      n42 = Bundle By Name(cluster=T2 {"min_deadband_floor"=0.0, "min_finetune_floor"=0.0, "dynamic_spindle_noise_scalar"=0.0, "filter_alpha"=0.0, "Vertical load (N)"=0.0, "Pulse delta"=0.0, "Fine Tune Zone"=0.0, "Max_pos_limit"=0.0, "Min_pos_limit"=0.0, "i_limit"=0.0, "Max Step Linit"=0.0, "Init Step"=0.0, "pct_scale"=0.0, "Deadband"=0.0, "Kd"=0.0, "Ki"=0.0, "Kp"=0.0, "Current Position"=0.0, "Set Load"=0.0, "Current Load"=0.0, "gFF Rot 7"={0.0, 0.0, 0.0}, "Bypass Load"=FALSE, "Enter ByPass Load"=0.0, "apply load"=FALSE} ("Value"), "Pulse delta"=w7, "gFF Rot 7"=w6) -> (w8:T2)
      n43 = property on="Property Node" class="Clust (strict)"(reference=w42, "Value"=w47) -> (reference out=w46:refnum<vi>, error out=w45:errorcluster)  [unwired: 1 in]
      n44 = property on="Property Node" class="Clust (strict)"(reference=w11, "Value"=w8) -> (reference out=w13:refnum<vi>, error out=w12:errorcluster)  [unwired: 1 in]
      n45 = Close Reference(reference=w46, error in (no error)=w45) -> (error out=w41:errorcluster)
      n46 = call "HEAVE WRITE FGV.vi"("Enum - Menu"=Heave_Write_enum."WRITE", "error in (no error)"=w41, "main ref"=w10) -> ("error out"=w68:errorcluster)  [unwired: 8 in]
      n47 = Close Reference(reference=w13, error in (no error)=w12) -> ()  [unwired: 1 out]
    }
    frame Error {
    }
  }
  "error out" <- w1
